vi "Start.vi"(8 "ErrorIn":errorcluster, 11 "DotNETCamIn":refnum<class "DotNETCam.lvclass">) -> (0 "ErrorOut":errorcluster, 3 "DotNETCamOut":refnum<class "DotNETCam.lvclass">)   [LabVIEW 2021, in "DotNETCam.lvclass"]
uses:
  DotNETCam.lvclass
  C:/Localdata/Projects/TriekselSoft/TriekselsoftApplicationFramework/Source/.Externals/Library_TAF/YActor/YActor.lvclass
  .Externals/Library_TAF/YActor/YActor.lvclass/YActor.ctl
  .Externals/Library_TAF/YActor/ExeCmd_sync.vi
  .Externals/Library_TAF/YActor/private/SendCommand.vi
  .Externals/Library_TAF/YActor/private/WaitForReply.vi
  .Externals/Library_TAF/YActor/private/CreateLocalVI.vi
  .Externals/Library_TAF/YActor/private/ExeuteInlineVI.vi
  .Externals/Library_TAF/YActor/private/GetRemoteVIRef.vi
  .Externals/Library_TAF/YActor/private/GetNameOfVI.vi
  .Externals/Library_TAF/YActor/QuickCast.vi
  .Externals/Library_TAF/YActor/private/VINameProperty.vi
  .Externals/Library_TAF/YActor/private/MessageCounter.vi
  .Externals/Library_TAF/YActor/InlineReferencePool.vi
  .Externals/Library_TAF/YActor/private/ExecuteVI.vi
  .Externals/Library_TAF/YActor/YActor.lvclass
  C:/Localdata/Projects/TriekselSoft/TriekselsoftApplicationFramework/Source/.Externals/Library_TAF/YAFTAF/YAFTAF.lvclass
  C:/Localdata/Projects/TriekselSoft/TriekselsoftApplicationFramework/Source/.Externals/Interface_UserInterface_IFrontPanel/IFrontPanel/IFrontPanel.lvclass
  C:/Localdata/Projects/TriekselSoft/TriekselsoftApplicationFramework/Source/.Externals/Interface_TAF_IInterface/IInterface/IInterface.lvclass
  C:/Localdata/Projects/TriekselSoft/TriekselsoftApplicationFramework/Source/.Externals/Interface_Object_ICreateDestroy/ICreateDestroy/ICreateDestroy.lvclass
  C:/Localdata/Projects/TriekselSoft/TriekselsoftApplicationFramework/Source/.Externals/Interface_Object_IPersistentData/IPersistentData/IPersistentData.lvclass
  C:/Localdata/Projects/TriekselSoft/TriekselsoftApplicationFramework/Source/.Externals/Interface_TAF_ITAFObject/ITAFObject/ITAFObject.lvclass
  C:/Localdata/Projects/TriekselSoft/TriekselsoftApplicationFramework/Source/YAFTAFObjects/DotNETCam/DotNETCam.lvclass
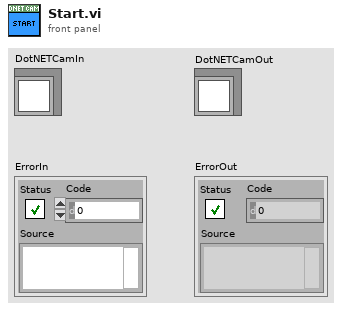
[diagram p1: front panel]
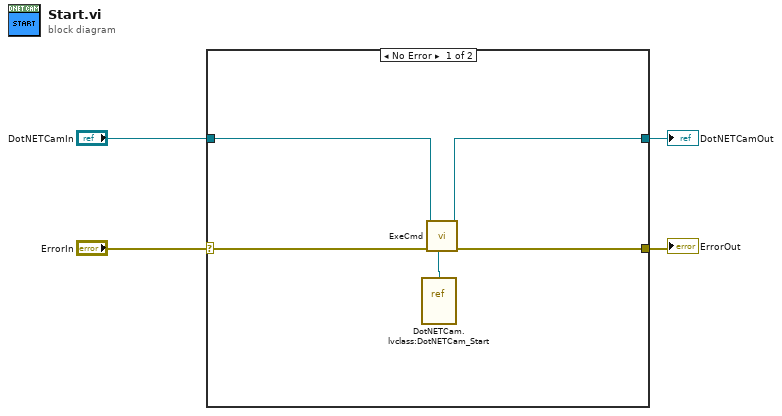
[diagram p0: block diagram]
diagram:
  n1 = case shown="No Error" "ErrorIn" {
    selector: "ErrorIn" -> [w9 w11]
    tunnel: [w8 w11] -> w3
    tunnel: [w5 w10] -> w1
    tunnel: "DotNETCamIn" -> [w6 w10]
    frame No Error {
      n2 = vi-ref "DotNETCam.lvclass:DotNETCam_Start.vi"() -> (w7:refnum<vi>)
      n3 = call-poly "ExeCmd.vi"("CmdVIRef"=w7, "ErrorIn"=w9, "YActorIn"=w6) -> ("ErrorOut"=w8:errorcluster, "YActorOut"=w5:refnum<class "DotNETCam.lvclass">)  [unwired: 6 in, 1 out]
    }
    frame Error {
    }
  }
  "ErrorOut" <- w3
  "DotNETCamOut" <- w1
